vi "Force control.vi"() -> ()   [LabVIEW 2021]
uses:
  <vilib>/Platform/TimedLoop/XDataNode/timing_clust.ctl
  <vilib>/Platform/TimedLoop/XDataNode/nitl_modes.ctl
  <vilib>/Platform/TimedLoop/XDataNode/wakeup.ctl
  <vilib>/DAQmx/write.llb/DAQmx Write (Digital Bool 1Line 1Point).vi
  <vilib>/DAQmx/write.llb/DAQmx Write (Analog DBL 1Chan 1Samp).vi
  <vilib>/DAQmx/create/channels.llb/DAQmx Create Channel (AI-Voltage-Basic).vi
  <vilib>/DAQmx/create/channels.llb/DAQmx Create Channel (DO-Digital Output).vi
  <vilib>/DAQmx/create/channels.llb/DAQmx Create Channel (AO-Voltage-Basic).vi
  <vilib>/DAQmx/miscellaneous.llb/DAQmx Fill In Error Info.vi
  <vilib>/addons/control/pid/pid.llb/PID (DBL).vi
  <vilib>/Platform/TimedLoop/XDataNode/XDataNode.xnode
  <vilib>/Platform/TimedLoop/XDataNode/XDNodeRunTimeDep.lvlib
  <vilib>/addons/control/pid/NI_PID_pid.lvlib
panel:
  out "Waveform Chart":cluster{"Filtered x":dbl, "Ref Force":dbl}(graph) caption="A"
  out "Total(V)":dbl
  in  "PID ON/OFF":bool
  in  "PID gains":T1={"proportional gain (Kc)"=0.3, "integral time (Ti, min)"=0.1, "derivative time (Td, min)"=0.0} {"derivative time (Td, min)" format="%.3f"; "integral time (Ti, min)" format="%.3f"; "proportional gain (Kc)" format="%.3f"}
  in  "Ref Force":dbl(slide) scale=0.0..40.0
  in  "Motor Enable":bool
  in  "stop":bool
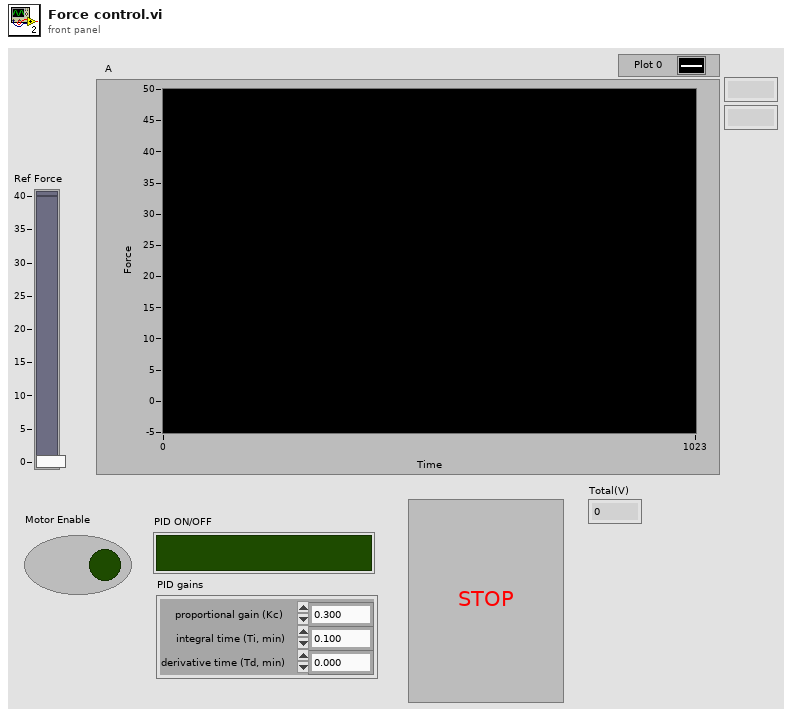
[diagram p1: front panel]
types:
  T1 = cluster{"proportional gain (Kc)":dbl, "integral time (Ti, min)":dbl, "derivative time (Td, min)":dbl}
  T2 = typedef "XDNodeRunTimeDep.lvlib/timing_clust.ctl" = cluster{"Expected End [f-1]":u64, "Actual End [f-1]":u64, "Finished Late? [f-1]":bool, "Expected End [i-1]":u64, "Actual End [i-1]":u64, "Finished Late? [i-1]":bool, "Expected Start [i]":u64, "Actual Start [i]":u64, "Expected Start [f]":u64, "Actual Start [f]":u64, "Source Name":string, "Structure Name":string, "Period":i64, "Deadline":i64, "Offset":i64, "Start":i64, "Priority":i32, "Timeout":i32, "Mode":T3, "Wakeup Reason":T4, "Error":errorcluster, "Source Type":string, "Secondary Source Type":string, "Global End Time":u64, "Global Start Time":u64, "Frame Duration":u64, "Iteration Duration":u64, "Assigned CPU":i32, "I/O Scan Engine Mode":u32}
  T3 = typedef "XDNodeRunTimeDep.lvlib/nitl_modes.ctl" = enum32{"No Change", "Process missed periods, maintain original phase", "Discard missed periods, maintain original phase", "Process missed periods, ignore original phase", "Discard missed periods, ignore original phase"}
  T4 = typedef "XDNodeRunTimeDep.lvlib/wakeup.ctl" = enum32{"Normal", "Aborted", "Asynchronous wakeup", "Timing source error", "Timed loop error", "Timeout"}
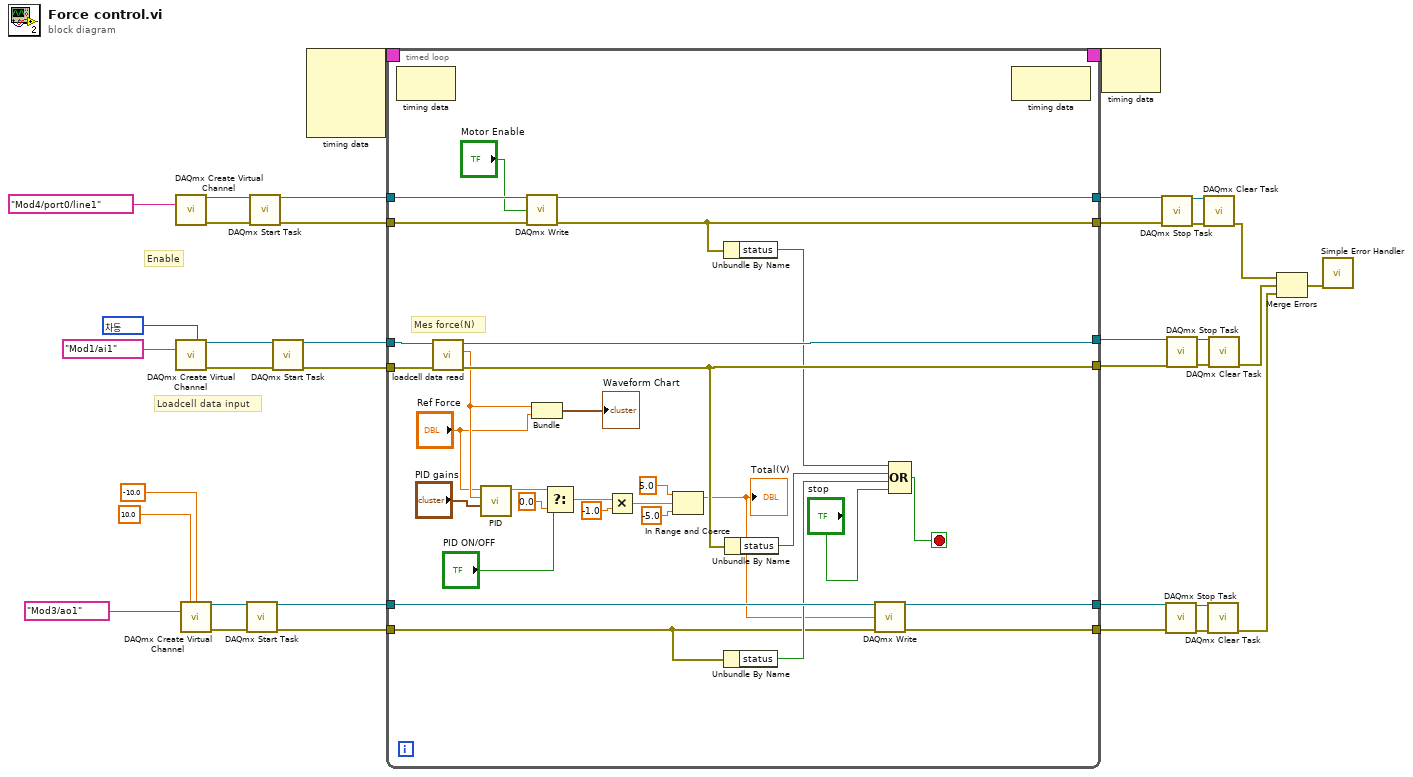
[diagram p0: block diagram]
diagram:
  w25 = 10106 items=["기본"=-1, "RSE"=10083, "NRSE"=10078, "차동"=10106, "유사 차동"=12529] ("input terminal configuration")
  # "Enable"
  # "Loadcell data input"
  n1 = call-poly <vilib>:"DAQmx Create Virtual Channel.vi"("lines"=tag "Mod4/port0/line1") -> ("task out"=w24:refnum<k21>, "error out"=w23:errorcluster)  [unwired: 13 in]
  n2 = call-poly <vilib>:"DAQmx Create Virtual Channel.vi"("input terminal configuration"=w25, "physical channels"=tag "Mod1/ai1") -> ("task out"=w33:refnum<k21>, "error out"=w32:errorcluster)  [unwired: 12 in]
  n3 = call-poly <vilib>:"DAQmx Create Virtual Channel.vi"("maximum value"=10.0, "minimum value"=-10.0, "physical channels"=tag "Mod3/ao1") -> ("task out"=w12:refnum<k21>, "error out"=w11:errorcluster)  [unwired: 11 in]
  n4 = call <vilib>:"DAQmx Start Task.vi"("task/channels in"=w12, "error in"=w11) -> ("task out"=w7:refnum<k21>, "error out"=w6:errorcluster)  [unwired: 12 in]
  n5 = call <vilib>:"DAQmx Start Task.vi"("task/channels in"=w24, "error in"=w23) -> ("task out"=w21:refnum<k21>, "error out"=w20:errorcluster)  [unwired: 12 in]
  n6 = call <vilib>:"DAQmx Start Task.vi"("task/channels in"=w33, "error in"=w32) -> ("task out"=w31:refnum<k21>, "error out"=w30:errorcluster)  [unwired: 12 in]
  n7 = node-c288() -> (w36:T2)  [unwired: 4 in]
  n8 = timed-loop {
    timing: w36 -> [_]
    timing-out: [_] -> w35
    tunnel: w31 -> [w67]
    tunnel: w30 -> [w66]
    tunnel: [w65] -> w26
    tunnel: [w64] -> w27
    tunnel: w21 -> [w61]
    tunnel: w20 -> [w60]
    tunnel: [w58] -> w17
    tunnel: [w57] -> w16
    tunnel: w7 -> [w55]
    tunnel: w6 -> [w50]
    tunnel: [w54] -> w3
    tunnel: [w53] -> w2
    stop <- w62 stop-if-true
    # "Mes force(N)"
    n9 = node-c288() -> ()  [unwired: 1 in, 1 out]
    n10 = call "loadcell data read.vi"("error in (no error)"=w66, "Refnum in"=w67) -> ("error out"=w64:errorcluster, "Filtered x"=w42:dbl, "Refnum out"=w65:refnum<k21>)  [unwired: 7 in]
    n11 = call-poly <vilib>:"PID.vi"("PID gains"="PID gains", "process variable"=w42, "setpoint"="Ref Force") -> ("output"=w48:dbl)  [unwired: 7 in, 1 out]
    n12 = call-poly <vilib>:"DAQmx Write.vi"("task/channels in"=w61, "data"="Motor Enable", "error in"=w60) -> ("task out"=w58:refnum<k21>, "error out"=w57:errorcluster)  [unwired: 10 in, 1 out]
    n13 = Bundle("Filtered x"=w42, "Ref Force"="Ref Force") -> (→"Waveform Chart":cluster{"Filtered x":dbl, "Ref Force":dbl})  [unwired: 1 in]
    n14 = Select(t=w48, s="PID ON/OFF", f=0.0) -> (s? t:f=w39:dbl)
    n15 = Multiply(x=w39, y=-1.0) -> (x*y=w37:dbl)
    n16 = In Range and Coerce(upper limit=5.0, x=w37, lower limit=-5.0) -> (coerced(x)=w43:dbl)  [unwired: 1 out]
    "Total(V)" <- w43
    n17 = Unbundle By Name(w57) -> ("status"=w56:bool)
    n18 = Unbundle By Name(w50) -> ("status"=w52:bool)
    n19 = Unbundle By Name(w64) -> ("status"=w63:bool)
    n20 = call-poly <vilib>:"DAQmx Write.vi"("task/channels in"=w55, "data"=w43, "error in"=w50) -> ("task out"=w54:refnum<k21>, "error out"=w53:errorcluster)  [unwired: 10 in, 1 out]
    n21 = Compound Arithmetic op=OR(w56, w63, w52, "stop") -> (w62:bool)
    n22 = node-c288() -> ()  [unwired: 1 in, 1 out]
  }
  n23 = node-c288(w35) -> ()  [unwired: 1 out]
  n24 = call <vilib>:"DAQmx Stop Task.vi"("task/channels in"=w17, "error in"=w16) -> ("task out"=w19:refnum<k21>, "error out"=w18:errorcluster)  [unwired: 12 in]
  n25 = call <vilib>:"DAQmx Stop Task.vi"("task/channels in"=w3, "error in"=w2) -> ("task out"=w5:refnum<k21>, "error out"=w4:errorcluster)  [unwired: 12 in]
  n26 = call <vilib>:"DAQmx Stop Task.vi"("task/channels in"=w26, "error in"=w27) -> ("task out"=w29:refnum<k21>, "error out"=w28:errorcluster)  [unwired: 12 in]
  n27 = call <vilib>:"DAQmx Clear Task.vi"("task in"=w19, "error in"=w18) -> ("error out"=w15:errorcluster)  [unwired: 13 in]
  n28 = call <vilib>:"DAQmx Clear Task.vi"("task in"=w5, "error in"=w4) -> ("error out"=w1:errorcluster)  [unwired: 13 in]
  n29 = call <vilib>:"DAQmx Clear Task.vi"("task in"=w29, "error in"=w28) -> ("error out"=w14:errorcluster)  [unwired: 13 in]
  n30 = Merge Errors(w15, w14, w1) -> (w13:errorcluster)
  n31 = call <vilib>:"Simple Error Handler.vi"("error in (no error)"=w13) -> ()  [unwired: 4 in, 5 out]
